vi "Leakage.vi"(0 "TSM context":T1, 5 "Pins and Pin Groups":tag[](array[tag]), 7 "Force Voltage (V)":dbl format="%#_13p", 9 "Current Limit (A)":dbl=2e-05 format="%#_13p", 12 "Aperture Time (s)":dbl=4e-06 format="%#_13p", 13 "Settling Time (s)":dbl=0.0005 format="%#_13p") -> (15 "error out":errorcluster)   [LabVIEW 2020]
doc: "Use this VI to perform a single leakage measurement using NI SMU(s) with the NI-DCPower driver or digital PPMU(s) with the NI-Digital Pattern Driver. The VI configures the instruments connected to the pins you specify, sources voltage on each pin, and measures the current on all pins simultaneously. You can provide input values to the VI to specify the voltage to source and the current limit for the leakage measurement.\n\nThe Leakage Test VI publishes the leakage current measurements for each pin. Configure test evaluations on the Tests tab of the Step Settings pane in TestStand to evaluate the results of these measurements."
uses:
  <vilib>/NI_TestStand_SemiconductorModule/NI_TestStand_Semiconductor_Module.lvlibp/PinMap/General/SemiconductorModuleContext.ctl
  <vilib>/NI_TestStand_SemiconductorModule/NI_TestStand_Semiconductor_Module.lvlibp/PinMap/General/NIInstrumentTypeIDs.ctl
  <instrlib>/niDCPower/nidcpower.llb/niDCPower Wait For Event - Event.ctl
  e564fa7b-be4c-4e15-afbe-3cc2524e3df0.vi
  5b1fb944-fc2a-48aa-b182-ef9cebfb7ebf.vi
  dc26616b-357a-4bf9-ae3c-3c5ac203ab79.vi
  99d4b74f-55e6-490b-b005-a31bc928c7d9.vi
  e564fa7b-be4c-4e15-afbe-3cc2524e3df0.vi/8545e684-78e7-4f2d-9f45-e9bff70177d8.vi
  e564fa7b-be4c-4e15-afbe-3cc2524e3df0.vi/c85ac437-d0e2-4ac4-855a-a47c4e00e2a5.vi
  e564fa7b-be4c-4e15-afbe-3cc2524e3df0.vi/c91900b9-8627-4539-964e-1e9f6389c2b2.vi
  e564fa7b-be4c-4e15-afbe-3cc2524e3df0.vi/8b096095-95d4-4f8d-a48e-81b6ba50300d.vi
  e564fa7b-be4c-4e15-afbe-3cc2524e3df0.vi/09f4c322-67db-4155-9942-2445e107da8c.vi
  5b1fb944-fc2a-48aa-b182-ef9cebfb7ebf.vi/bc2f0c86-5130-4572-b970-c21e3763abb5.vi
  5b1fb944-fc2a-48aa-b182-ef9cebfb7ebf.vi/bd0dd02f-133f-4cd2-8df3-7561b4b2536e.vi
  5b1fb944-fc2a-48aa-b182-ef9cebfb7ebf.vi/19e6d49f-1b60-46e1-9391-1dfed84695f2.vi
  5b1fb944-fc2a-48aa-b182-ef9cebfb7ebf.vi/486752ee-8f30-4a63-a088-6cbd4480e54b.vi
  Common/Instrument Control/Digital/SubVIs/SSC Digital Calculate Per-Site Per-Pin to Per-Instrument LUT.vi
  dc26616b-357a-4bf9-ae3c-3c5ac203ab79.vi/7ab91422-1a66-4814-9877-4eb2634f872c.vi
  dc26616b-357a-4bf9-ae3c-3c5ac203ab79.vi/78867d26-a5ff-4ac0-84e1-08aa210c9386.vi
  99d4b74f-55e6-490b-b005-a31bc928c7d9.vi/4689e3c1-66eb-4ef1-9eb6-df5da4ed0aa5.vi
  99d4b74f-55e6-490b-b005-a31bc928c7d9.vi/1b0eca36-914e-49e1-9c38-e654956cdac7.vi
  99d4b74f-55e6-490b-b005-a31bc928c7d9.vi/90f49b17-a1f6-4a07-917b-c7890f56ae33.vi
  99d4b74f-55e6-490b-b005-a31bc928c7d9.vi/8dccb768-e49e-474e-bfb0-f94b19b49205.vi
  Common/Instrument Control/Shared SubVIs/Channel List to Pins.vi
  Common/Instrument Control/Shared SubVIs/Trim Whitespace [Inlined].vi
  <vilib>/NI_TestStand_SemiconductorModule/NI_TestStand_Semiconductor_Module.lvlibp/PinMap/Digital Pattern/PinQueryContext/DigitalPatternPinQueryContext.lvclass
  C:/Program Files/National Instruments/LabVIEW 2020/vi.lib/NI_TestStand_SemiconductorModule/NI_TestStand_Semiconductor_Module.lvlibp/PinMap/PinQueryContext/MultipleSessionPinQueryContext.lvclass
  <vilib>/NI_TestStand_SemiconductorModule/NI_TestStand_Semiconductor_Module.lvlibp/PinMap/PinQueryContext/MultiplePinMultipleSessionQueryContext/MultiplePinMultipleSessionQueryContext.lvclass
  C:/Program Files/National Instruments/LabVIEW 2020/vi.lib/NI_TestStand_SemiconductorModule/NI_TestStand_Semiconductor_Module.lvlibp/PinMap/PinQueryContext/PinQueryContext.lvclass
  Common/Instrument Control/DCPower/SSC DCPower/Measure/SSC DCPower Configure Settings Array.vi
  Common/Instrument Control/DCPower/SSC DCPower/SSC DCPower Configure Measurements.vi
  Common/Instrument Control/DCPower/SSC DCPower/Source/Constant Voltage/SSC DCPower Force Voltage Array Symmetric Limits.vi
  Common/Instrument Control/Digital/SSC Digital/PPMU/SSC Digital PPMU Configure Aperture Time.vi
  Common/Instrument Control/Digital/SSC Digital/PPMU/SSC Digital PPMU Source Voltage.vi
  Common/Instrument Control/DCPower/SSC DCPower/Triggers and Events/SSC DCPower Wait for Event.vi
  Common/Instrument Control/DCPower/SSC DCPower/SSC DCPower Measure.vi
  <vilib>/NI_TestStand_SemiconductorModule/NI_TestStand_Semiconductor_Module.lvlibp/PinMap/General/Publish/PublishDataDouble1D.vi
  <vilib>/NI_TestStand_SemiconductorModule/NI_TestStand_Semiconductor_Module.lvlibp/PinMap/General/Publish/PublishDataDouble2D.vi
  <vilib>/NI_TestStand_SemiconductorModule/NI_TestStand_Semiconductor_Module.lvlibp
  C:/Program Files/National Instruments/LabVIEW 2020/vi.lib/NI_TestStand_SemiconductorModule/NI_TestStand_Semiconductor_Module.lvlibp/PinMap/PinQueryContext/MultiplePinMultipleSessionQueryContext/MultiplePinMultipleSessionQueryContext.lvclass
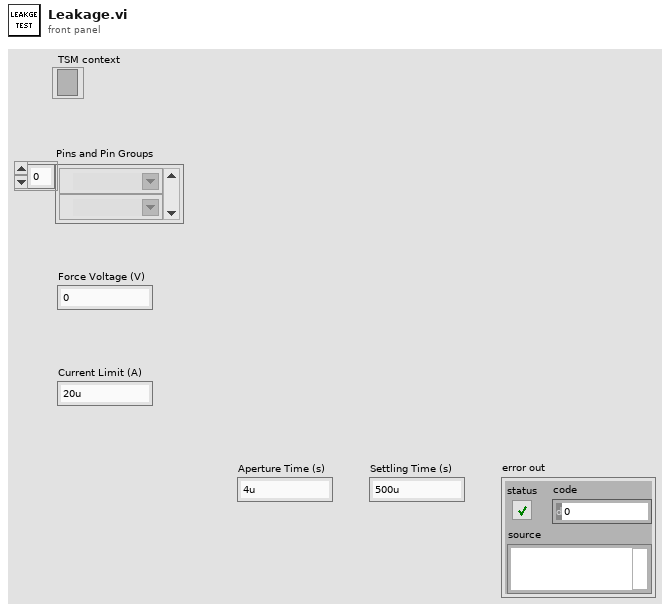
[diagram p1: front panel]
types:
  T1 = typedef "NI_TestStand_Semiconductor_Module.lvlibp/SemiconductorModuleContext.ctl" = refnum<k7>
  T2 = typedef "niDCPower Wait For Event - Event.ctl" = i32
  T3 = typedef "NI_TestStand_Semiconductor_Module.lvlibp/NIInstrumentTypeIDs.ctl" = string
  T4 = typedef "NI_TestStand_Semiconductor_Module.lvlibp/TSM_Pin.ctl" = tag
  T5 = typedef "TSM SSC Digital.ctl" = cluster{"Pin Query Context":refnum<class "DigitalPatternPinQueryContext.lvclass">, "SSC":T6[], "Site Numbers":i32[], "Pins":tag[]}
  T6 = typedef "SSC Digital.ctl" = cluster{"Session":refnum<k15>, "Channel List":string, "Site List":string}
  T7 = typedef "TSM SSC DCPower.ctl" = cluster{"Pin Query Context":refnum<class "MultiplePinMultipleSessionQueryContext.lvclass">, "SSC":T8[], "Site Numbers":i32[], "Pins":T9[], "Pins Expanded":T11[]}
  T8 = typedef "SSC DCPower.ctl" = cluster{"Session":refnum<k15>, "Chan":string, "Channel List":string}
  T9 = typedef "TSM Pin Information.ctl" = cluster{"Pin":tag, "Type":T10, "Count":i32}
  T10 = typedef "TSM Pin Type Identifier.ctl" = enum8{"DUT Pin", "System Pin", "Pin Group", "Not Determined"}
  T11 = typedef "TSM Expanded Pin Information.ctl" = cluster{"Pin":tag, "Type":T10, "Index":i32}
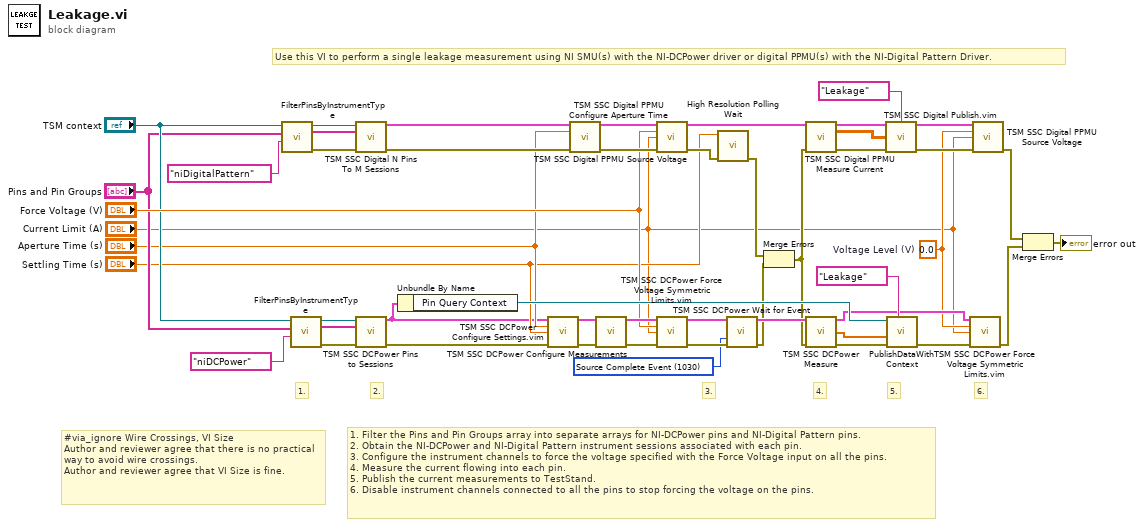
[diagram p0: block diagram]
diagram:
  w6 = 0.0  # Voltage Level (V)
  w7 = T2 1030 items=["Source Complete Event"=1030, "Measure Complete Event"=1031, "Sequence Iteration Complete Event"=1032, "Sequence Engine Done Event"=1033, "Pulse Complete Event"=1051, "Ready For Pulse Trigger Event"=1052] ("Event")
  # "#via_ignore Wire Crossings, VI Size\nAuthor and reviewer agree that there is no practical way to avoid wire crossings.\nAuthor and reviewer agree that VI Size is fine."
  # "6."
  # "5."
  # "4."
  # "3."
  # "2."
  # "1."
  # "1. Filter the Pins and Pin Groups array into separate arrays for NI-DCPower pins and NI-Digital Pattern pins.\n2. Obtain the NI-DCPower and NI-Digital Pattern instrument sessions associated with each pin.\n3. Configure the instrument channels to force the voltage specified with the Force Voltage input on all the pins.\n4. Measure the current flowing into each pin.\n5. Publish the current measurements to TestStand.\n6. Disable instrument channels connected to all the pins to stop forcing the voltage on the pins."
  # "Use this VI to perform a single leakage measurement using NI SMU(s) with the NI-DCPower driver or digital PPMU(s) with the NI-Digital Pattern Driver."
  n1 = call <vilib>:"FilterPinsByInstrumentType.vi"("Instrument Type Id"=T3 "niDigitalPattern", "Pins"="Pins and Pin Groups", "Semiconductor Module Context"="TSM context") -> ("error out"=w18:errorcluster, "Filtered Pins"=w15:T4[], "Semiconductor Module Context Out"=w16:T1)  [unwired: 6 in]
  n2 = call <vilib>:"FilterPinsByInstrumentType.vi"("Instrument Type Id"=T3 "niDCPower", "Pins"="Pins and Pin Groups", "Semiconductor Module Context"="TSM context") -> ("error out"=w46:errorcluster, "Filtered Pins"=w47:T4[], "Semiconductor Module Context Out"=w48:T1)  [unwired: 6 in]
  n3 = call "TSM SSC Digital N Pins To M Sessions.vi"("TSM context"=w16, "Pins"=w15, "error in"=w18) -> ("Digital TSM Out"=w33:T5, "error out"=w31:errorcluster)  [unwired: 11 in]
  n4 = call "TSM SSC DCPower Pins to Sessions.vi"("TSM context"=w48, "Pins"=w47, "error in"=w46) -> ("DCPower TSM Out"=w1:T7, "error out"=w21:errorcluster)  [unwired: 11 in]
  n5 = Unbundle By Name(w1) -> ("Pin Query Context"=w32:refnum<class "MultiplePinMultipleSessionQueryContext.lvclass">)
  n6 = call "TSM SSC DCPower Configure Settings.vim"("DCPower TSM in"=w1, "Aperture Time"="Aperture Time (s)", "Source Delay (s)"="Settling Time (s)", "error in"=w21) -> ("DCPower TSM out"=w44:T7, "error out"=w22:errorcluster)  [unwired: 10 in]
  n7 = call "TSM SSC Digital PPMU Configure Aperture Time.vi"("Digital TSM In"=w33, "Aperture Time (s)"="Aperture Time (s)", "error in"=w31) -> ("Digital TSM Out"=w41:T5, "error out"=w42:errorcluster)  [unwired: 11 in]
  n8 = call "TSM SSC DCPower Configure Measurements.vi"("DCPower SSC in"=w44, "error in"=w22) -> ("DCPower SSC out"=w43:T7, "error out"=w23:errorcluster)  [unwired: 12 in]
  n9 = call "TSM SSC Digital PPMU Source Voltage.vi"("Digital TSM In"=w41, "Voltage Level (V)"="Force Voltage (V)", "Current Limit Range (A)"="Current Limit (A)", "error in"=w42) -> ("Digital TSM Out"=w30:T5, "error out"=w45:errorcluster)  [unwired: 10 in]
  n10 = call "TSM SSC DCPower Force Voltage Symmetric Limits.vim"("DCPower TSM in"=w43, "Voltage Level (V)"="Force Voltage (V)", "Current Limit (A)"="Current Limit (A)", "error in"=w23) -> ("DCPower TSM out"=w9:T7, "error out"=w24:errorcluster)  [unwired: 10 in]
  n11 = call <vilib>:"High Resolution Polling Wait.vi"("error in (no error)"=w45, "seconds to wait"="Settling Time (s)") -> ("error out"=w5:errorcluster)  [unwired: 9 in]
  n12 = call "TSM SSC DCPower Wait for Event.vi"("DCPower TSM in"=w9, "Event"=w7, "error in"=w24) -> ("DCPower TSM out"=w8:T7, "error out"=w4:errorcluster)  [unwired: 11 in]
  n13 = Merge Errors(w5, w4) -> (w3:errorcluster)
  n14 = call "TSM SSC Digital PPMU Measure Current.vi"("Digital TSM In"=w30, "error in"=w3) -> ("Digital TSM out"=w38:T5, "Per-Site Per-Pin Measurements (A)"=w37:dbl[][], "error out"=w39:errorcluster)  [unwired: 11 in]
  n15 = call "TSM SSC DCPower Measure.vi"("DCPower TSM in"=w8, "error in"=w3) -> ("DCPower TSM out"=w12:T7, "Current Measurements (A)"=w34:dbl[], "error out"=w40:errorcluster)  [unwired: 10 in, 1 out]
  n16 = call "TSM SSC Digital Publish.vim"("Digital TSM In"=w38, "Published Data Id"=tag "Leakage", "Data to Publish"=w37, "error in (no error)"=w39) -> ("Digital TSM Out"=w29:T5, "error out"=w28:errorcluster)  [unwired: 10 in]
  n17 = call-poly <vilib>:"PublishDataWithContext.vi"("Published Data Id"=tag "Leakage", "error in (no error)"=w40, "Data In"=w34, "Pin Query Context"=w32) -> ("error out"=w25:errorcluster)  [unwired: 6 in, 1 out]
  n18 = call "TSM SSC DCPower Force Voltage Symmetric Limits.vim"("DCPower TSM in"=w12, "Voltage Level (V)"=w6, "Current Limit (A)"="Current Limit (A)", "error in"=w25) -> ("error out"=w26:errorcluster)  [unwired: 10 in, 1 out]
  n19 = call "TSM SSC Digital PPMU Source Voltage.vi"("Digital TSM In"=w29, "Voltage Level (V)"=w6, "Current Limit Range (A)"="Current Limit (A)", "error in"=w28) -> ("error out"=w27:errorcluster)  [unwired: 10 in, 1 out]
  n20 = Merge Errors(w27, w26) -> (→"error out":errorcluster)
